vi "Setup Example.vi"(8 "error in (no error)":errorcluster, 11 "CCD in":refnum<class "CCD.lvclass">) -> (0 "error out":errorcluster, 2 "Module Was Already Running?":bool, 3 "CCD out":refnum<class "CCD.lvclass">)   [LabVIEW 2023]
uses:
  CCD.lvclass
  DeviceManager/DeviceManager.lvlib
panel:
  # "Connector Pane"
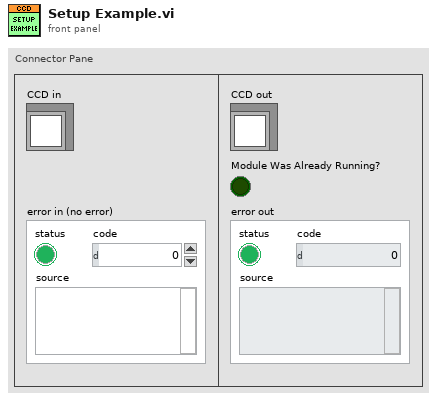
[diagram p1: front panel]
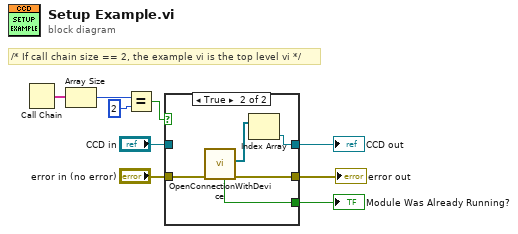
[diagram p0: block diagram]
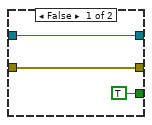
[diagram p2: hidden frame]
diagram:
  # "/* If call chain size == 2, the example vi is the top level vi */"
  n1 = Call Chain() -> (call chain=w4:string[])
  n2 = Array Size(array=w4) -> (size(s)=w5:i32)
  n3 = Equal?(x=w5, y=2) -> (x = y?=w7:bool)
  n4 = case shown="True" w7 {
    tunnel: [w12 w15] -> w8
    tunnel: "CCD in" -> [w12 _]
    tunnel: [TRUE ("Module Was Already Running?") w16] -> w3
    tunnel: "error in (no error)" -> [w11 w14]
    tunnel: [w11 w13] -> w1
    frame False {
    }
    frame True {
      n5 = call "OpenConnectionWithDevice.vi"("error in"=w14) -> ("error out"=w13:errorcluster, "CCDs"=w17:refnum<class "CCD.lvclass">[], "Module Was Already Running?"=w16:bool)  [unwired: 6 in, 2 out]
      n6 = Index Array(array=w17) -> (element=w15:refnum<class "CCD.lvclass">)  [unwired: 1 in]
    }
  }
  "CCD out" <- w8
  "error out" <- w1
  "Module Was Already Running?" <- w3
